vi "Calculate Score.vi"(11 "Remaining string":string[](array[string])) -> (3 "Score":u64)   [LabVIEW 2019, in "Day 10.lvlib"]
uses:
  Day 10.lvlib
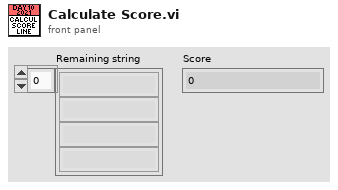
[diagram p1: front panel]
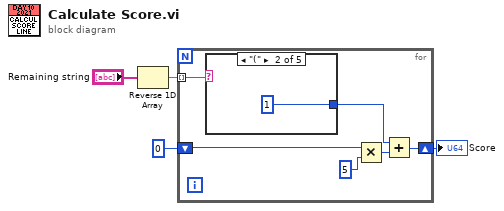
[diagram p0: block diagram]
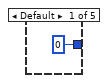
[diagram p2: hidden frame]
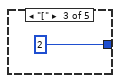
[diagram p3: hidden frame]
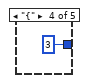
[diagram p4: hidden frame]
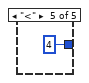
[diagram p5: hidden frame]
diagram:
  n1 = Reverse 1D Array(array="Remaining string") -> (reversed array=w2:string[])
  n2 = for {
    tunnel: w2 -> [w10] mode=indexing
    shift-right: [w8] -> w4
    shift-left: u64 0 -> [w9]
    n3 = case shown="\"(\"" w10 {
      tunnel: [u64 0 u64 1 u64 2 u64 3 u64 4] -> w7
      frame Default {
      }
      frame "(" {
      }
      frame "[" {
      }
      frame "{" {
      }
      frame "<" {
      }
    }
    n4 = Multiply(x=w9, y=u64 5) -> (x*y=w5:u64)
    n5 = Add(x=w7, y=w5) -> (x+y=w8:u64)
  }
  "Score" <- w4
